vi "example.vi"() -> ()   [LabVIEW 2017]
uses:
  Source/Control Scripting/Control Population Settings.ctl
  Source/Advanced Variant Tools.lvlib
panel:
  out "String":string
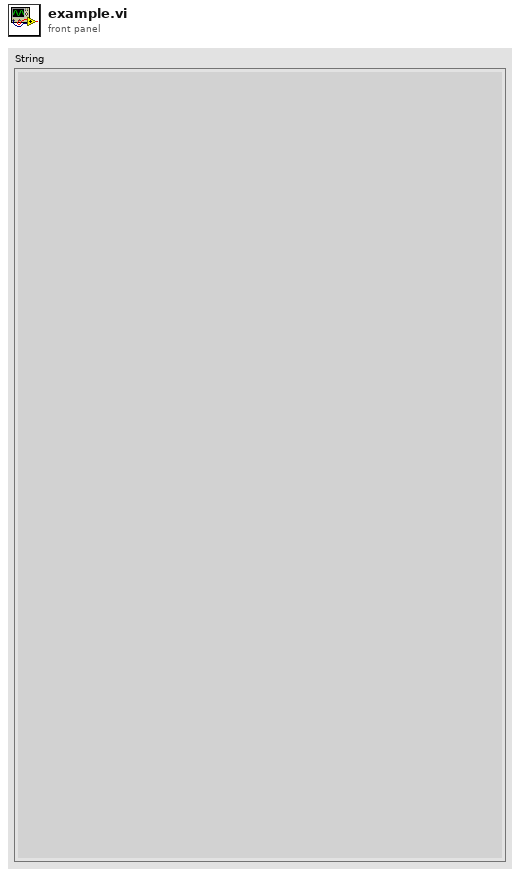
[diagram p1: front panel]
types:
  T1 = typedef "Advanced Variant Tools.lvlib/Control Population Settings.ctl" = enum16{"Set Values as Default", "Populate Only", "None"}
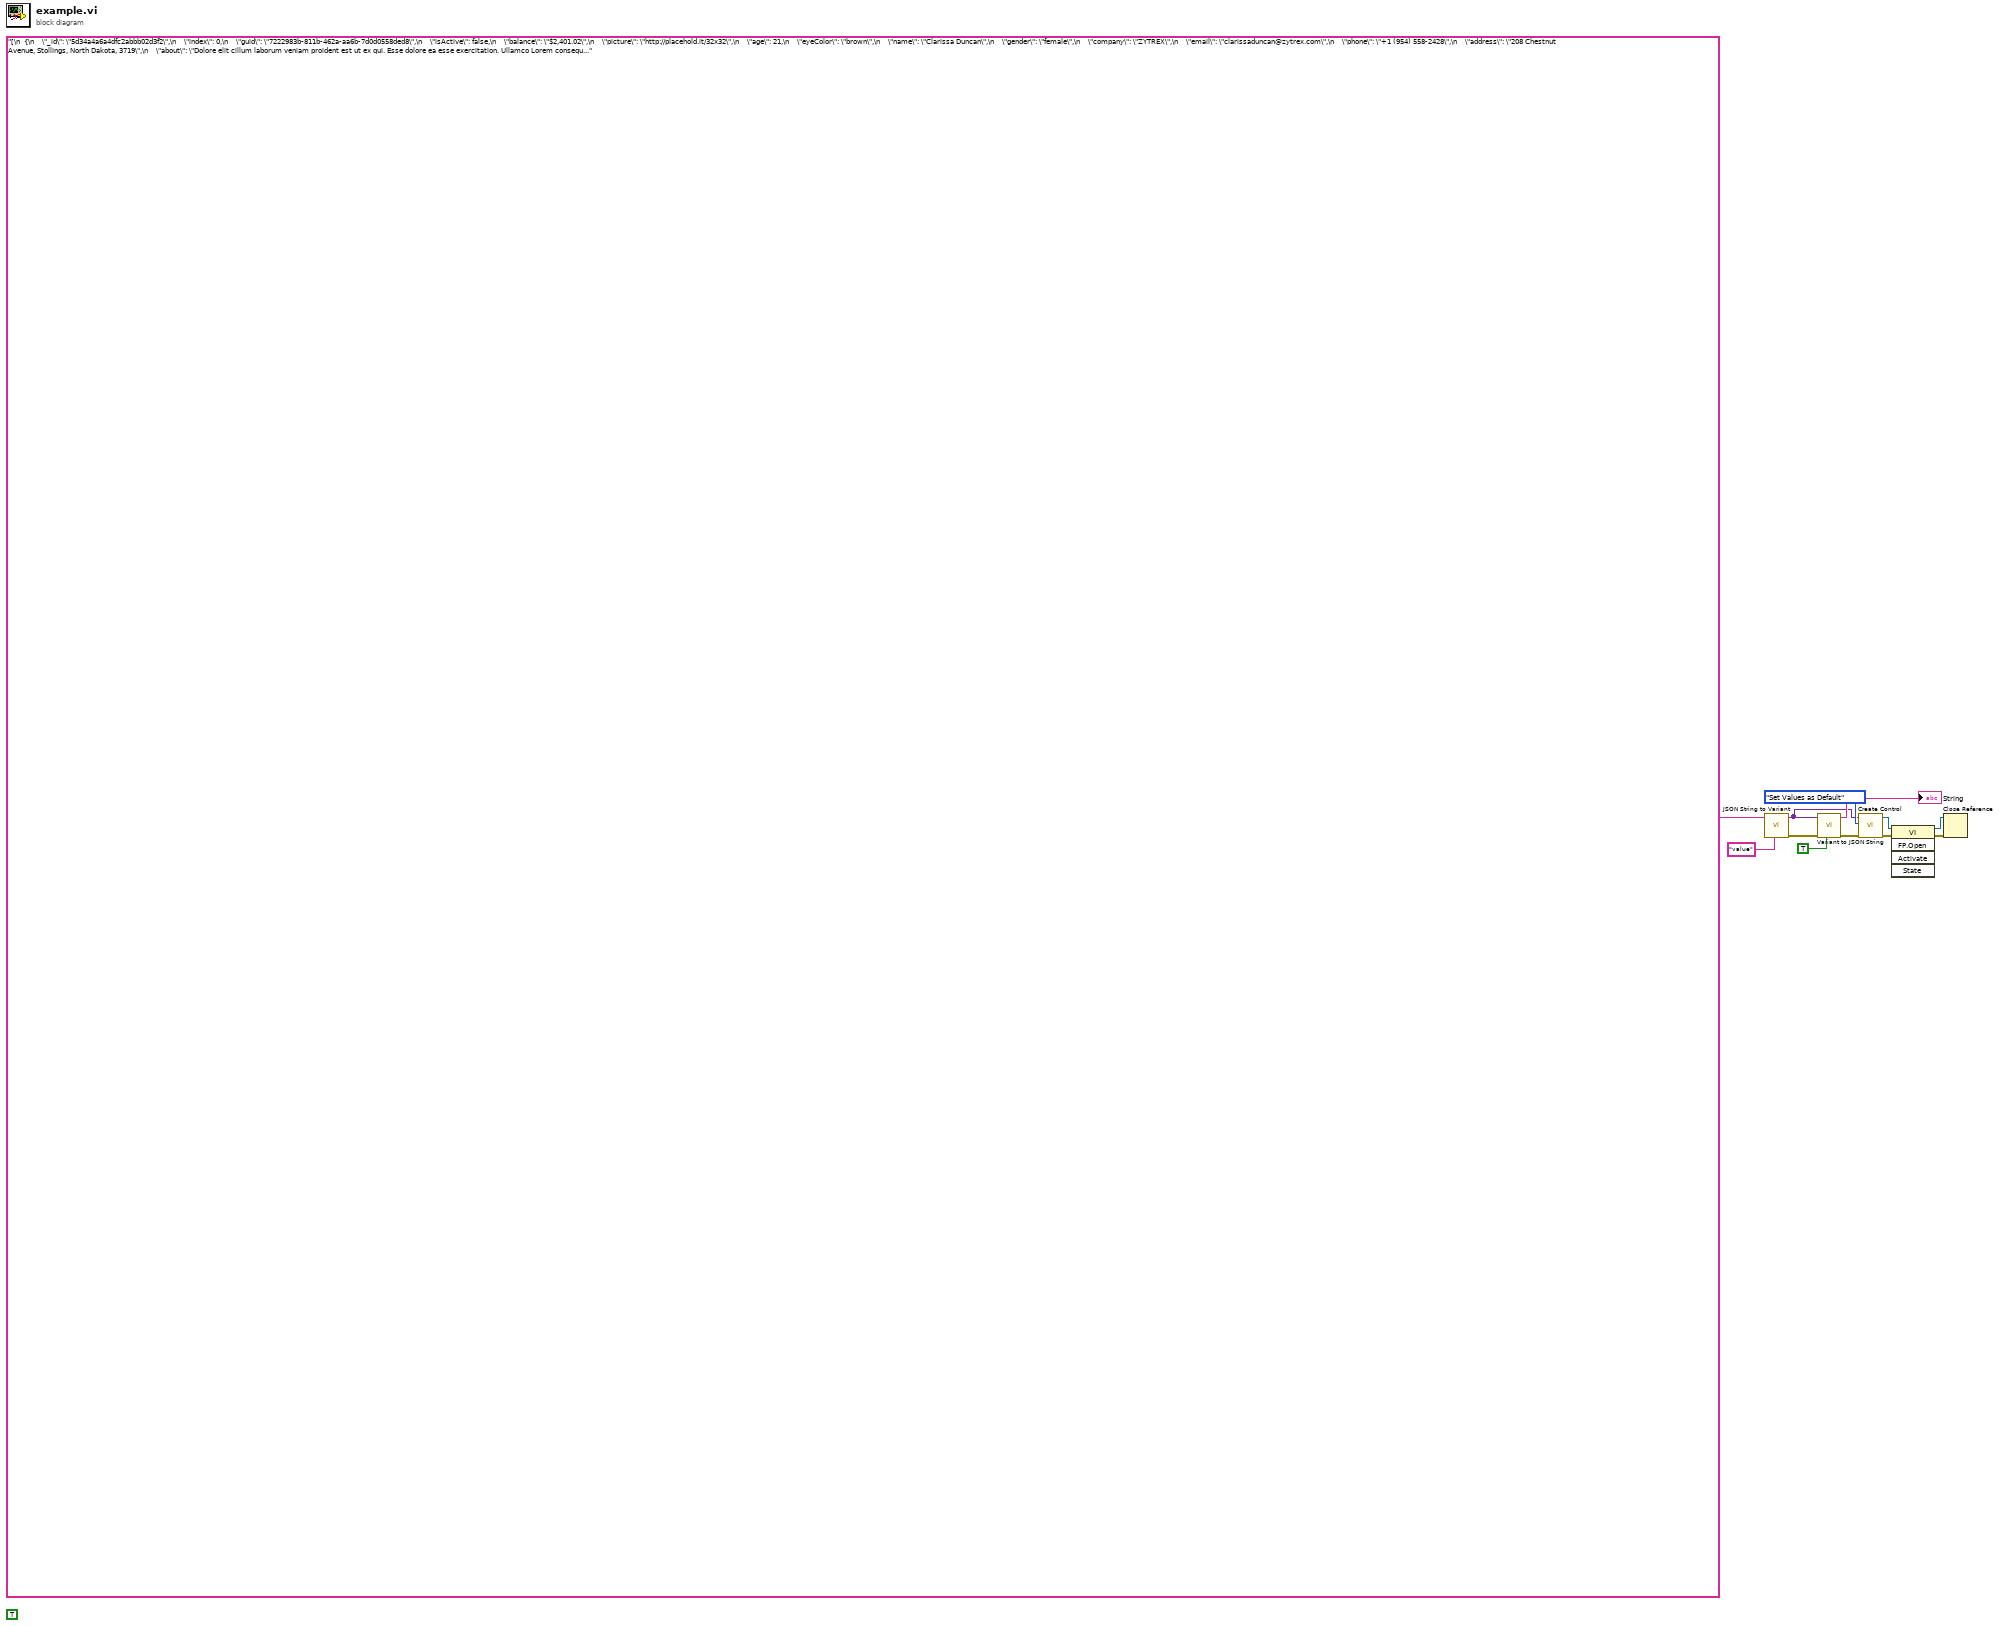
[diagram p0: block diagram]
diagram:
  (unwired) TRUE ("add values to arrays")
  n1 = call "JSON String to Variant.vi"("Top-Level Control Name"="value", "JSON String"="[\n  {\n    \"_id\": \"5d34a4a6a4dfc2abbb02d3f2\",\n    \"index\": 0,\n    \"guid\": \"7222983b-811b-462a-aa6b-7d0d0558ded8\",\n    \"isActive\": false,\n    \"balance\": \"$2,401.02\",\n    \"picture\": \"http://placehold.it/32x32\",\n    \"age\": 21,\n    \"eyeColor\": \"brown\",\n    \"name\": \"Clarissa Duncan\",\n    \"gender\": \"female\",\n    \"company\": \"ZYTREX\",\n    \"email\": \"clarissaduncan@zytrex.com\",\n    \"phone\": \"+1 (954) 558-2428\",\n    \"address\": \"208 Chestnut Avenue, Stollings, North Dakota, 3719\",\n    \"about\": \"Dolore elit cillum laborum veniam proident est ut ex qui. Esse dolore ea esse exercitation. Ullamco Lorem consequat pariatur dolore pariatur culpa veniam sit cillum id. Occaecat cillum consequat mollit cupidatat dolore ea pariatur labore in quis officia pariatur ullamco adipisicing. Id cillum minim sit minim aute cillum ut anim eu ad sint do. Et ut laborum enim elit non enim labore ipsum ut dolore culpa labore.\\r\\n\",\n    \"registered\": \"2015-04-21T11:40:42 +05:00\",\n    \"latitude\": -28.650392,\n    \"longitude\": -179.505084,\n    \"tags\": [\n      \"fugiat\",\n      \"voluptate\",\n      \"reprehenderit\",\n      \"ea\",\n      \"exercitation\",\n      \"ea\",\n      \"velit\"\n    ],\n    \"friends\": [\n      {\n        \"id\": 0,\n        \"name\": \"Landry Navarro\"\n      },\n      {\n        \"id\": 1,\n        \"name\": \"Bridges Briggs\"\n      },\n      {\n        \"id\": 2,\n        \"name\": \"Miller Singleton\"\n      }\n    ],\n    \"greeting\": \"Hello, Clarissa Duncan! You have 6 unread messages.\",\n    \"favoriteFruit\": \"strawberry\"\n  },\n  {\n    \"_id\": \"5d34a4a6348a28400566aa21\",\n    \"index\": 1,\n    \"guid\": \"3877b229-616e-44b1-8def-97efa3c0481b\",\n    \"isActive\": true,\n    \"balance\": \"$1,081.97\",\n    \"picture\": \"http://placehold.it/32x32\",\n    \"age\": 33,\n    \"eyeColor\": \"blue\",\n    \"name\": \"Buckley Travis\",\n    \"gender\": \"male\",\n    \"company\": \"KENGEN\",\n    \"email\": \"buckleytravis@kengen.com\",\n    \"phone\": \"+1 (825) 534-2551\",\n    \"address\": \"369 Newkirk Placez, Goldfield, Indiana, 5871\",\n    \"about\": \"Adipisicing ipsum nostrud id exercitation ex. Eiusmod officia culpa voluptate exercitation qui irure amet non exercitation. Veniam laboris amet eu adipisicing fugiat. Dolore proident dolor laboris tempor ea enim. Dolor labore in quis sunt voluptate adipisicing ipsum velit Lorem enim ipsum aute nulla.\\r\\n\",\n    \"registered\": \"2019-05-15T12:13:38 +05:00\",\n    \"latitude\": -73.258256,\n    \"longitude\": 95.52394,\n    \"tags\": [\n      \"mollit\",\n      \"proident\",\n      \"occaecat\",\n      \"magna\",\n      \"amet\",\n      \"eiusmod\",\n      \"est\"\n    ],\n    \"friends\": [\n      {\n        \"id\": 0,\n        \"name\": \"Hale Patrick\"\n      },\n      {\n        \"id\": 1,\n        \"name\": \"Roxanne David\"\n      },\n      {\n        \"id\": 2,\n        \"name\": \"Harper Mendez\"\n      }\n    ],\n    \"greeting\": \"Hello, Buckley Travis! You have 2 unread messages.\",\n    \"favoriteFruit\": \"apple\"\n  },\n  {\n    \"_id\": \"5d34a4a6d7c6434910007a45\",\n    \"index\": 2,\n    \"guid\": \"22820776-661a-4eb8-826e-86f07020e74d\",\n    \"isActive\": true,\n    \"balance\": \"$2,233.62\",\n    \"picture\": \"http://placehold.it/32x32\",\n    \"age\": 34,\n    \"eyeColor\": \"green\",\n    \"name\": \"Luella Williamson\",\n    \"gender\": \"female\",\n    \"company\": \"CALCU\",\n    \"email\": \"luellawilliamson@calcu.com\",\n    \"phone\": \"+1 (816) 544-3518\",\n    \"address\": \"515 Sullivan Place, Kent, Connecticut, 8246\",\n    \"about\": \"Enim consequat amet adipisicing voluptate consectetur eiusmod consequat dolor adipisicing dolore ad ullamco excepteur. Officia tempor proident anim ad est proident. Ullamco laboris ea ad officia quis consectetur enim dolor minim esse tempor velit.\\r\\n\",\n    \"registered\": \"2019-07-12T08:50:58 +05:00\",\n    \"latitude\": 4.79475,\n    \"longitude\": 81.818394,\n    \"tags\": [\n      \"labore\",\n      \"ut\",\n      \"do\",\n      \"voluptate\",\n      \"minim\",\n      \"ea\",\n      \"amet\"\n    ],\n    \"friends\": [\n      {\n        \"id\": 0,\n        \"name\": \"Melisa Mcleod\"\n      },\n      {\n        \"id\": 1,\n        \"name\": \"Patrice Mcclure\"\n      },\n      {\n        \"id\": 2,\n        \"name\": \"Hahn Whitehead\"\n      }\n    ],\n    \"greeting\": \"Hello, Luella Williamson! You have 5 unread messages.\",\n    \"favoriteFruit\": \"banana\"\n  }\n]") -> ("error out"=w3:errorcluster, "JSON Value out"=w4:variant)  [unwired: 8 in]
  n2 = call "Variant to JSON String.vi"("pretty print? (F)"=TRUE, "error in (no error)"=w3, "JSON Value in"=w4) -> ("error out"=w2:errorcluster, "String"=→"String":string)  [unwired: 7 in]
  n3 = call "Create Control.vi"("error in (no error)"=w2, 10:Control_Population_Settings."Set Values as Default", "Variant in"=w4) -> ("error out"=w1:errorcluster, "Control VI Reference"=w9:refnum<vi>)  [unwired: 7 in]
  n4 = invoke class="VI" method="FP.Open"(reference=w9, error in=w1) -> (reference out=w8:refnum<vi>, error out=w7:errorcluster)  [unwired: 3 in, 3 out]
  n5 = Close Reference(reference=w8, error in (no error)=w7) -> ()  [unwired: 1 out]
